vi "未命名 1.vi"   [LabVIEW 2011]
uses:
  <vilib>/addons/database/Connection.llb/DB Tools Open Connec (String).vi
types:
  T1 = typedef "NI_Database_API.lvlib/Conn ObjectReference.ctl" = refnum<k1>
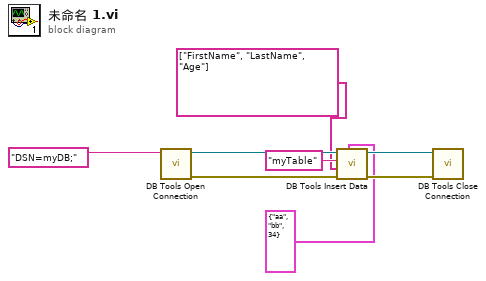
[diagram p0: block diagram]
diagram:
  n1 = call-poly <vilib>:"DB Tools Open Connection.vi"("connection information"="DSN=myDB;" ("ConnectionString")) -> ("error out"=w5:errorcluster, "connection reference"=w6:T1)  [unwired: 7 in]
  n2 = call <vilib>:"DB Tools Insert Data.vi"("data"=cluster{"字符串":string, "字符串 2":string, "数值":i32} {"字符串"="aa", "字符串 2"="bb", "数值"=34} ("簇"), "error in (no error)"=w5, "columns"=string[] ["FirstName", "LastName", "Age"], "table"="myTable", "connection reference"=w6) -> ("error out"=w7:errorcluster, "connection reference out"=w4:T1)  [unwired: 5 in]
  n3 = call <vilib>:"DB Tools Close Connection.vi"("error in (no error)"=w7, "connection reference"=w4) -> ()  [unwired: 5 in, 1 out]
